vi "Close.vi"(8 "error in":errorcluster, 11 "Voltage Actual Value in":refnum<class "Voltage Actual Value.lvclass">) -> (0 "error out":errorcluster, 3 "Voltage Actual Value out":refnum<class "Voltage Actual Value.lvclass">)   [LabVIEW 2023, in "Voltage Actual Value.lvclass"]
uses:
  Voltage Actual Value.lvclass
  Parents/Actual Value/Actual Value.lvclass
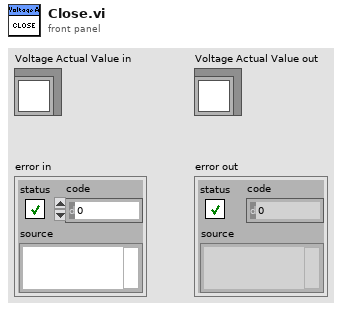
[diagram p1: front panel]
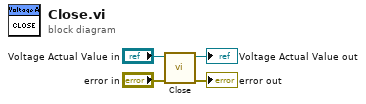
[diagram p0: block diagram]
diagram:
  n1 = call-parent "Close.vi"("error in"="error in", "Actual Value in"="Voltage Actual Value in") -> ("error out"=→"error out":errorcluster, "Actual Value out"=→"Voltage Actual Value out":refnum<class "Voltage Actual Value.lvclass">)  [unwired: 8 in]
